vi "Invoke Node (XNET UDP Socket).vi"   [LabVIEW 2018]
doc: "Methods in this node can be used with the XNET UDP Socket VIs."
uses:
  <resource>/objmgr/xnet.rc
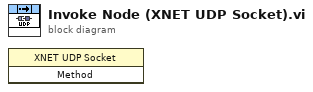
[diagram p0: block diagram]
diagram:
  n1 = invoke class="XNET UDP Socket" method=#-1() -> ()  [unwired: 3 in, 3 out]
